vi "Dequeue.vi"(8 "error in (no error)":errorcluster, 11 "Message Queue in":refnum<queue>) -> (0 "error out":errorcluster, 1 "Message Data":variant, 2 "Message":T1, 3 "Message Queue out":refnum<queue>)   [LabVIEW 2024]
uses:
  Message Cluster.ctl
  Message.ctl
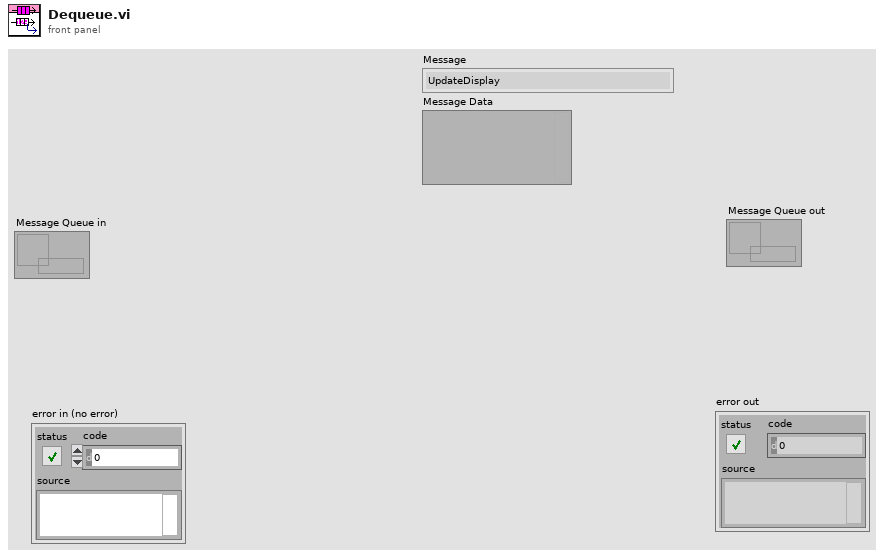
[diagram p1: front panel]
types:
  T1 = typedef "Message.ctl" = enum16{"UpdateDisplay", "Run Washing", "Exit", "Slider run", "Checking wash step", "Continuing washing", "Waiting for slider movement", "Initialize"}
  T2 = typedef "Message Cluster.ctl" = cluster{"Message":T1, "Message Data":variant}
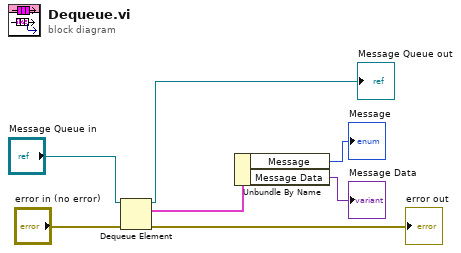
[diagram p0: block diagram]
diagram:
  n1 = Dequeue Element(queue="Message Queue in", error in (no error)="error in (no error)") -> (queue out=→"Message Queue out":refnum<queue>, element=w3:T2, error out=→"error out":errorcluster)  [unwired: 1 in, 1 out]
  n2 = Unbundle By Name(w3) -> ("Message"=→"Message":T1, "Message Data"=→"Message Data":variant)
